vi "計算時間測試.vi"() -> ()   [LabVIEW 2015]
panel:
  in  "Numeric":i32=10000
  out "noref":u32
  out "ref":u32
  out "x+y 2":i32
  out "x+y":i32
  in  "Numeric 50":i32
  in  "Numeric 49":i32
  in  "Numeric 48":i32
  in  "Numeric 47":i32
  in  "Numeric 46":i32
  in  "Numeric 45":i32
  in  "Numeric 44":i32
  in  "Numeric 43":i32
  in  "Numeric 42":i32
  in  "Numeric 41":i32
  in  "Numeric 40":i32
  in  "Numeric 39":i32
  in  "Numeric 38":i32
  in  "Numeric 37":i32
  in  "Numeric 36":i32
  in  "Numeric 35":i32
  in  "Numeric 34":i32
  in  "Numeric 33":i32
  in  "Numeric 32":i32
  in  "Numeric 31":i32
  in  "Numeric 30":i32
  in  "Numeric 29":i32
  in  "Numeric 28":i32
  in  "Numeric 27":i32
  in  "Numeric 26":i32
  in  "Numeric 25":i32
  in  "Numeric 24":i32
  in  "Numeric 23":i32
  in  "Numeric 22":i32
  in  "Numeric 21":i32
  in  "Numeric 20":i32
  in  "Numeric 19":i32
  in  "Numeric 18":i32
  in  "Numeric 17":i32
  in  "Numeric 16":i32
  in  "Numeric 15":i32
  in  "Numeric 14":i32
  in  "Numeric 13":i32
  in  "Numeric 12":i32
  in  "Numeric 11":i32
  in  "Numeric 10":i32
  in  "Numeric 9":i32
  in  "Numeric 8":i32
  in  "Numeric 7":i32
  in  "Numeric 6":i32
  in  "Numeric 5":i32
  in  "Numeric 4":i32
  in  "Numeric 3":i32
  in  "Numeric 2":i32
  in  "Numeric 1":i32
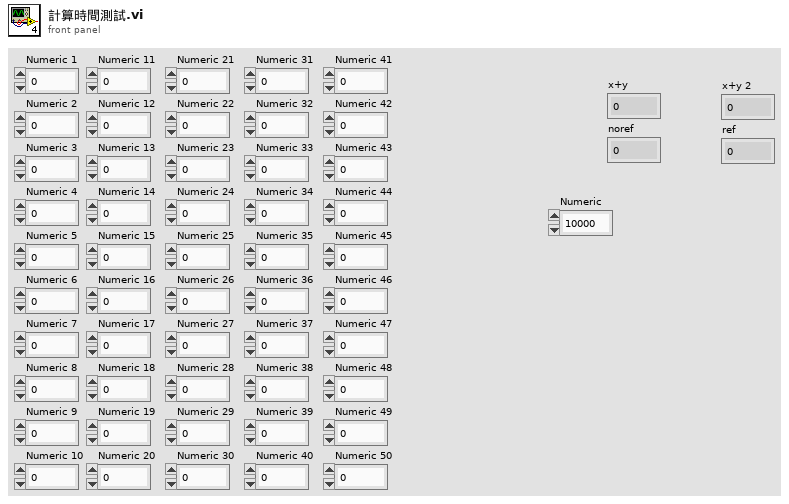
[diagram p1: front panel]
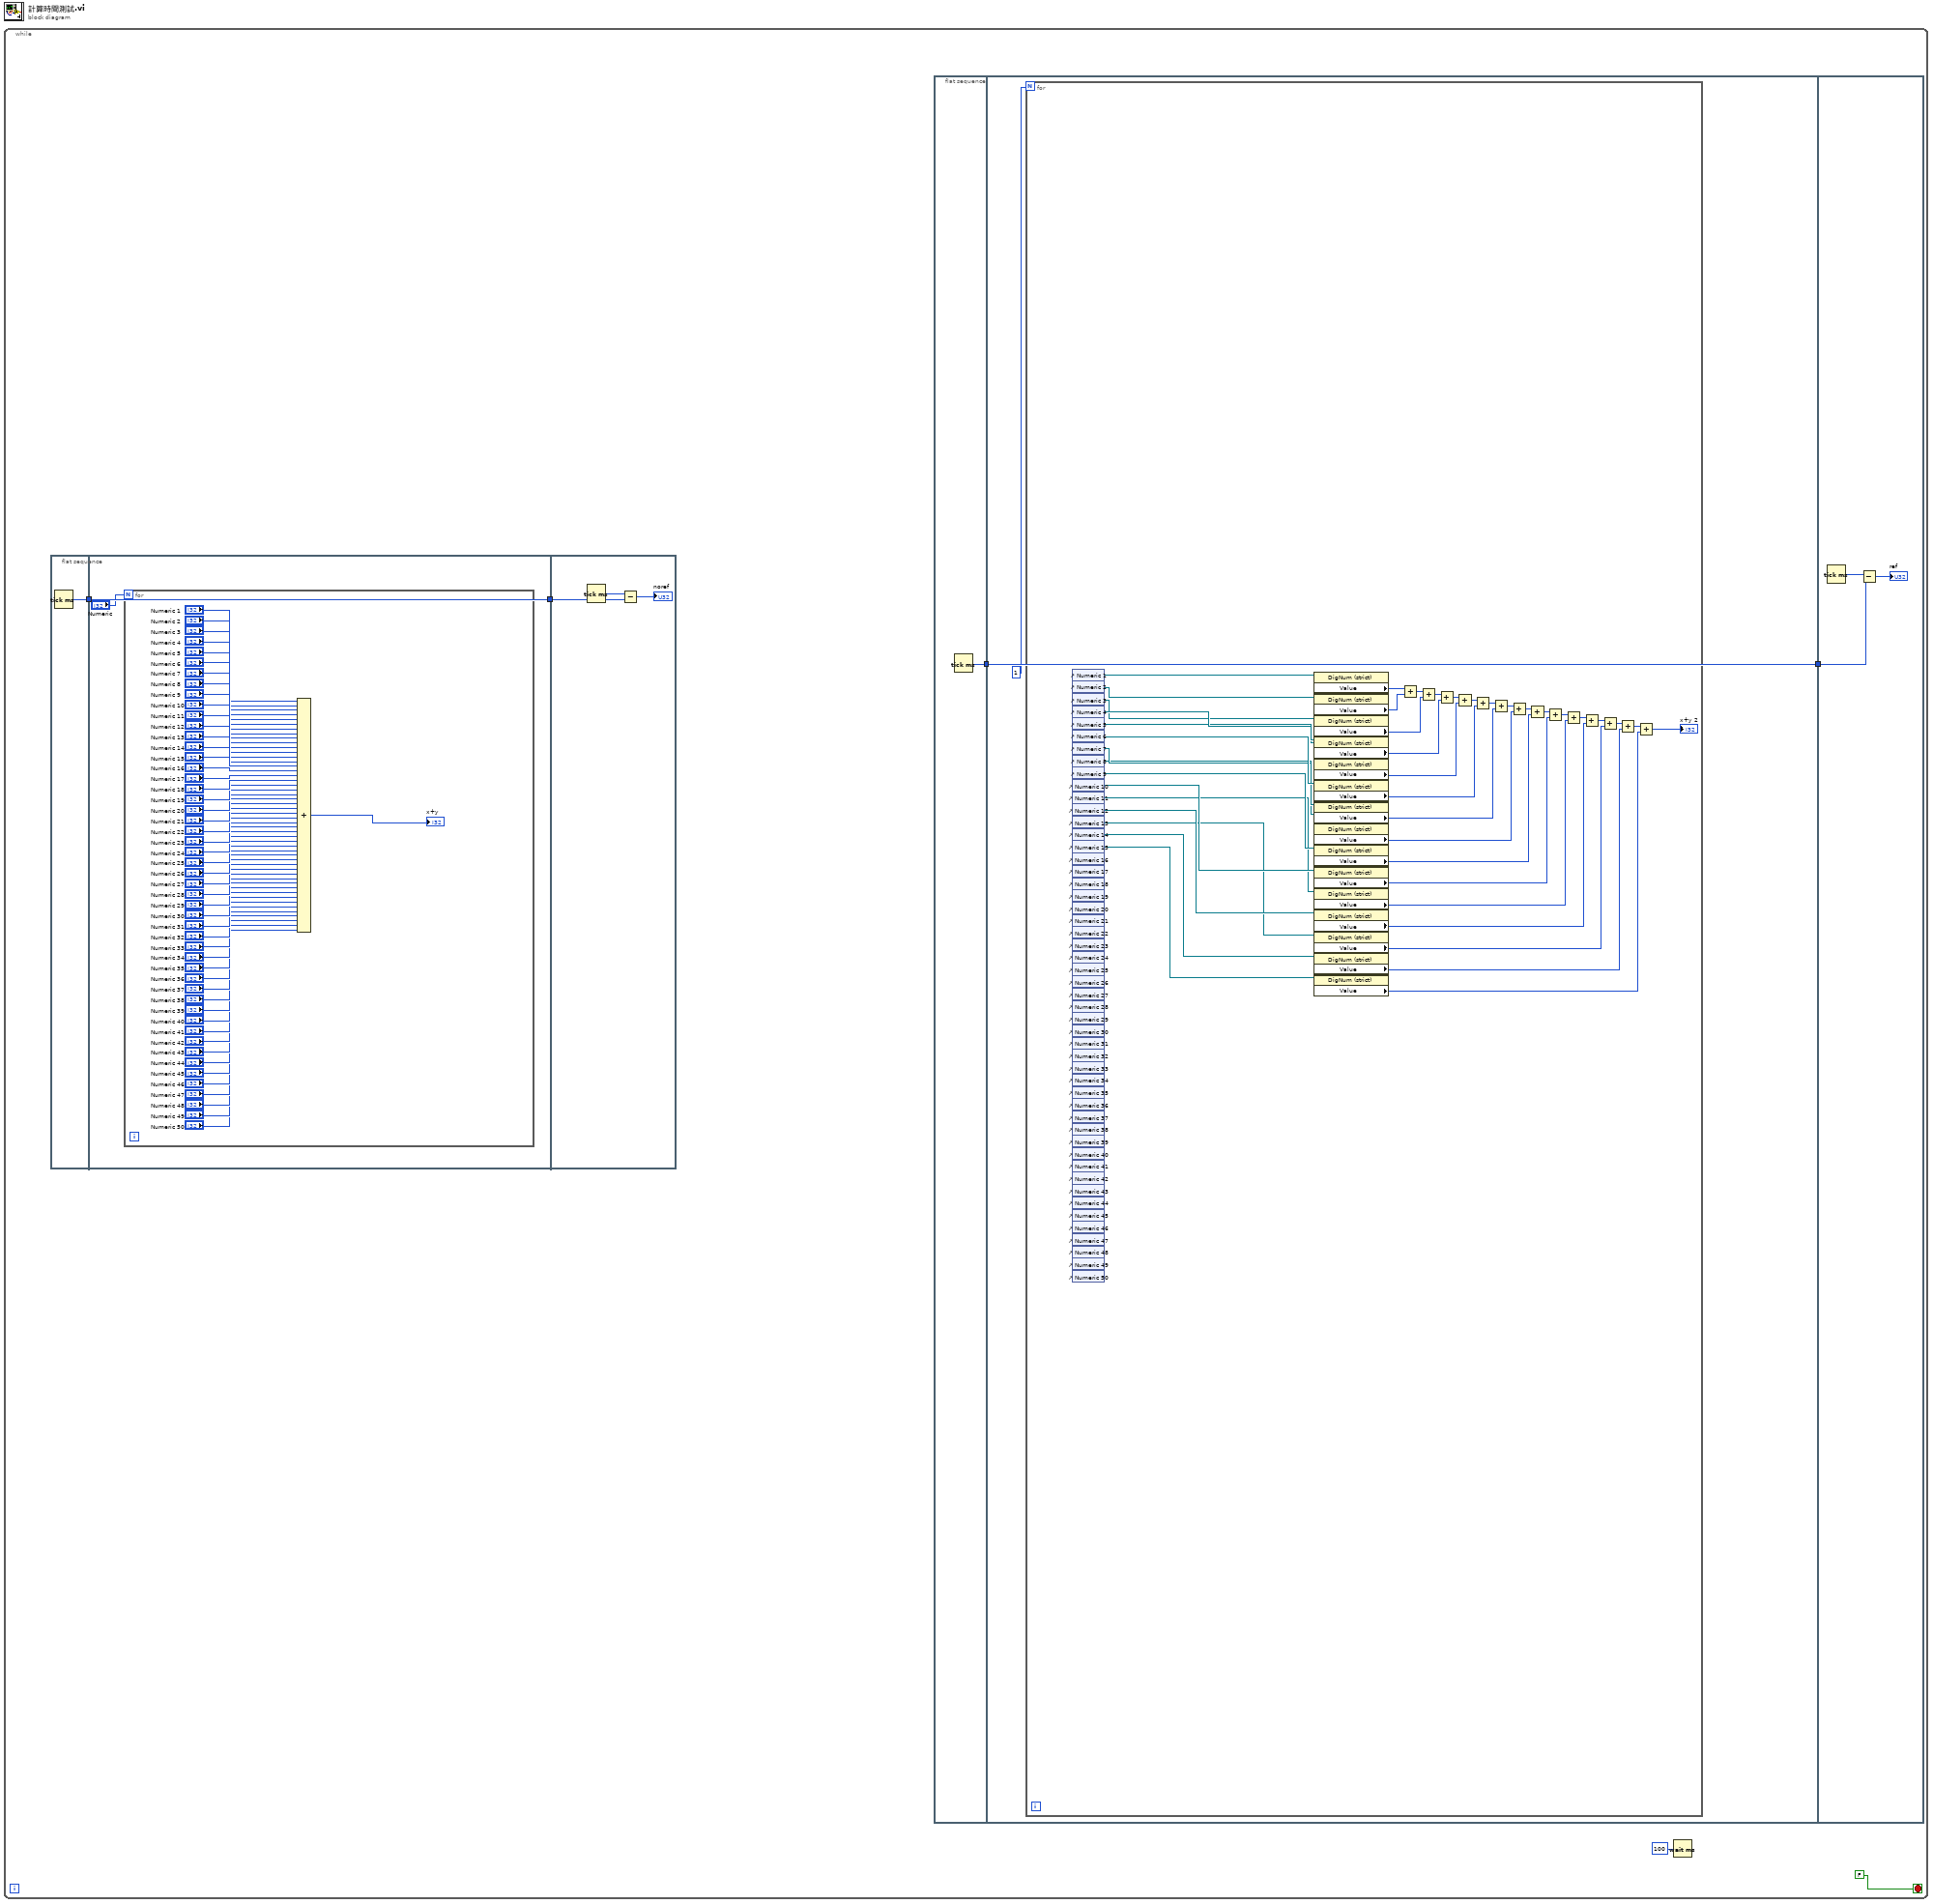
[diagram p0: block diagram]
diagram:
  n1 = while {
    stop <- FALSE stop-if-true
    n2 = flat-sequence {
      tunnel: [w7] -> w4
      tunnel: [w9] -> w3
      tunnel: w4 -> [w9]
      tunnel: w3 -> [w61]
      frame #0 {
        n3 = Tick Count (ms)() -> (millisecond timer value=w7:u32)
      }
      frame #1 {
        n4 = for {
          N: "Numeric" -> [_]
          n5 = Compound Arithmetic op=ADD("Numeric 1", "Numeric 2", "Numeric 3", "Numeric 4", "Numeric 5", "Numeric 6", "Numeric 7", "Numeric 8", "Numeric 9", "Numeric 10", "Numeric 11", "Numeric 12", "Numeric 13", "Numeric 14", "Numeric 15", "Numeric 16", "Numeric 17", "Numeric 18", "Numeric 19", "Numeric 20", "Numeric 21", "Numeric 22", "Numeric 23", "Numeric 24", "Numeric 25", "Numeric 26", "Numeric 27", "Numeric 28", "Numeric 29", "Numeric 30", "Numeric 31", "Numeric 32", "Numeric 33", "Numeric 34", "Numeric 35", "Numeric 36", "Numeric 37", "Numeric 38", "Numeric 39", "Numeric 40", "Numeric 41", "Numeric 42", "Numeric 43", "Numeric 44", "Numeric 45", "Numeric 46", "Numeric 47", "Numeric 48", "Numeric 49", "Numeric 50") -> (→"x+y":i32)
        }
      }
      frame #2 {
        n6 = Tick Count (ms)() -> (millisecond timer value=w63:u32)
        n7 = Subtract(x=w63, y=w61) -> (x-y=→"noref":u32)
      }
    }
    n8 = flat-sequence {
      tunnel: [w64] -> w6
      tunnel: [w66] -> w5
      tunnel: w6 -> [w66]
      tunnel: w5 -> [w112]
      frame #0 {
        n9 = Tick Count (ms)() -> (millisecond timer value=w64:u32)
      }
      frame #1 {
        n10 = for {
          N: 1 -> [_]
          n11 = control-ref of="Numeric 1"() -> (w67:refnum<vi>)
          n12 = control-ref of="Numeric 2"() -> (w110:refnum<vi>)
          n13 = control-ref of="Numeric 3"() -> (w100:refnum<vi>)
          n14 = control-ref of="Numeric 4"() -> (w109:refnum<vi>)
          n15 = control-ref of="Numeric 5"() -> (w108:refnum<vi>)
          n16 = control-ref of="Numeric 6"() -> (w107:refnum<vi>)
          n17 = control-ref of="Numeric 7"() -> (w106:refnum<vi>)
          n18 = control-ref of="Numeric 8"() -> (w105:refnum<vi>)
          n19 = control-ref of="Numeric 9"() -> (w104:refnum<vi>)
          n20 = control-ref of="Numeric 10"() -> (w103:refnum<vi>)
          n21 = control-ref of="Numeric 11"() -> (w102:refnum<vi>)
          n22 = control-ref of="Numeric 12"() -> (w101:refnum<vi>)
          n23 = control-ref of="Numeric 13"() -> (w99:refnum<vi>)
          n24 = control-ref of="Numeric 14"() -> (w98:refnum<vi>)
          n25 = control-ref of="Numeric 15"() -> (w97:refnum<vi>)
          n26 = control-ref of="Numeric 16"() -> ()  [unwired: 1 out]
          n27 = control-ref of="Numeric 17"() -> ()  [unwired: 1 out]
          n28 = control-ref of="Numeric 18"() -> ()  [unwired: 1 out]
          n29 = control-ref of="Numeric 19"() -> ()  [unwired: 1 out]
          n30 = control-ref of="Numeric 20"() -> ()  [unwired: 1 out]
          n31 = control-ref of="Numeric 21"() -> ()  [unwired: 1 out]
          n32 = control-ref of="Numeric 22"() -> ()  [unwired: 1 out]
          n33 = control-ref of="Numeric 23"() -> ()  [unwired: 1 out]
          n34 = control-ref of="Numeric 24"() -> ()  [unwired: 1 out]
          n35 = control-ref of="Numeric 25"() -> ()  [unwired: 1 out]
          n36 = control-ref of="Numeric 26"() -> ()  [unwired: 1 out]
          n37 = control-ref of="Numeric 27"() -> ()  [unwired: 1 out]
          n38 = control-ref of="Numeric 28"() -> ()  [unwired: 1 out]
          n39 = control-ref of="Numeric 29"() -> ()  [unwired: 1 out]
          n40 = control-ref of="Numeric 30"() -> ()  [unwired: 1 out]
          n41 = control-ref of="Numeric 31"() -> ()  [unwired: 1 out]
          n42 = control-ref of="Numeric 32"() -> ()  [unwired: 1 out]
          n43 = control-ref of="Numeric 33"() -> ()  [unwired: 1 out]
          n44 = control-ref of="Numeric 34"() -> ()  [unwired: 1 out]
          n45 = control-ref of="Numeric 35"() -> ()  [unwired: 1 out]
          n46 = control-ref of="Numeric 36"() -> ()  [unwired: 1 out]
          n47 = control-ref of="Numeric 37"() -> ()  [unwired: 1 out]
          n48 = control-ref of="Numeric 38"() -> ()  [unwired: 1 out]
          n49 = control-ref of="Numeric 39"() -> ()  [unwired: 1 out]
          n50 = control-ref of="Numeric 40"() -> ()  [unwired: 1 out]
          n51 = control-ref of="Numeric 41"() -> ()  [unwired: 1 out]
          n52 = control-ref of="Numeric 42"() -> ()  [unwired: 1 out]
          n53 = control-ref of="Numeric 43"() -> ()  [unwired: 1 out]
          n54 = control-ref of="Numeric 44"() -> ()  [unwired: 1 out]
          n55 = control-ref of="Numeric 45"() -> ()  [unwired: 1 out]
          n56 = control-ref of="Numeric 46"() -> ()  [unwired: 1 out]
          n57 = control-ref of="Numeric 47"() -> ()  [unwired: 1 out]
          n58 = control-ref of="Numeric 48"() -> ()  [unwired: 1 out]
          n59 = control-ref of="Numeric 49"() -> ()  [unwired: 1 out]
          n60 = control-ref of="Numeric 50"() -> ()  [unwired: 1 out]
          n61 = property class="DigNum (strict)"(reference=w67) -> ("Value"=w83:i32)  [unwired: 1 in, 2 out]
          n62 = property class="DigNum (strict)"(reference=w110) -> ("Value"=w82:i32)  [unwired: 1 in, 2 out]
          n63 = property class="DigNum (strict)"(reference=w100) -> ("Value"=w81:i32)  [unwired: 1 in, 2 out]
          n64 = property class="DigNum (strict)"(reference=w109) -> ("Value"=w80:i32)  [unwired: 1 in, 2 out]
          n65 = property class="DigNum (strict)"(reference=w108) -> ("Value"=w79:i32)  [unwired: 1 in, 2 out]
          n66 = property class="DigNum (strict)"(reference=w107) -> ("Value"=w78:i32)  [unwired: 1 in, 2 out]
          n67 = property class="DigNum (strict)"(reference=w106) -> ("Value"=w77:i32)  [unwired: 1 in, 2 out]
          n68 = property class="DigNum (strict)"(reference=w105) -> ("Value"=w76:i32)  [unwired: 1 in, 2 out]
          n69 = property class="DigNum (strict)"(reference=w104) -> ("Value"=w75:i32)  [unwired: 1 in, 2 out]
          n70 = property class="DigNum (strict)"(reference=w103) -> ("Value"=w74:i32)  [unwired: 1 in, 2 out]
          n71 = property class="DigNum (strict)"(reference=w102) -> ("Value"=w73:i32)  [unwired: 1 in, 2 out]
          n72 = property class="DigNum (strict)"(reference=w101) -> ("Value"=w72:i32)  [unwired: 1 in, 2 out]
          n73 = property class="DigNum (strict)"(reference=w99) -> ("Value"=w71:i32)  [unwired: 1 in, 2 out]
          n74 = property class="DigNum (strict)"(reference=w98) -> ("Value"=w70:i32)  [unwired: 1 in, 2 out]
          n75 = property class="DigNum (strict)"(reference=w97) -> ("Value"=w69:i32)  [unwired: 1 in, 2 out]
          n76 = Add(x=w83, y=w82) -> (x+y=w91:i32)
          n77 = Add(x=w91, y=w81) -> (x+y=w96:i32)
          n78 = Add(x=w96, y=w80) -> (x+y=w95:i32)
          n79 = Add(x=w95, y=w79) -> (x+y=w94:i32)
          n80 = Add(x=w94, y=w78) -> (x+y=w93:i32)
          n81 = Add(x=w93, y=w77) -> (x+y=w92:i32)
          n82 = Add(x=w92, y=w76) -> (x+y=w84:i32)
          n83 = Add(x=w84, y=w75) -> (x+y=w90:i32)
          n84 = Add(x=w90, y=w74) -> (x+y=w89:i32)
          n85 = Add(x=w89, y=w73) -> (x+y=w88:i32)
          n86 = Add(x=w88, y=w72) -> (x+y=w87:i32)
          n87 = Add(x=w87, y=w71) -> (x+y=w86:i32)
          n88 = Add(x=w86, y=w70) -> (x+y=w85:i32)
          n89 = Add(x=w85, y=w69) -> (x+y=→"x+y 2":i32)
        }
      }
      frame #2 {
        n90 = Tick Count (ms)() -> (millisecond timer value=w113:u32)
        n91 = Subtract(x=w113, y=w112) -> (x-y=→"ref":u32)
      }
    }
    n92 = Wait (ms)(milliseconds to wait=u32 100) -> ()  [unwired: 1 out]
  }
